vi "Close.vi"(6 "Priority (F)":bool, 8 "error in (no error)":errorcluster, 11 "Data":variant) -> (0 "error out":errorcluster)   [LabVIEW 2020, in "Controller.lvlib"]
uses:
  Private Controls/Element.ctl
  Private Controls/Module Action.ctl
  Controller.lvlib
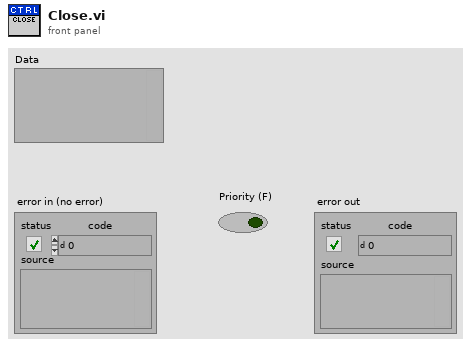
[diagram p1: front panel]
types:
  T1 = typedef "Controller.lvlib/Module Action.ctl" = enum16{"Initialise Module", "Connect", "Setup", "Pause", "Start", "Search Network", "Get Local", "Process Results", "Stop", "Show Match", "Show Full", "Get UI Refs", "Wait: Time Elapsed", "Error", "Exit"}
  T2 = typedef "Controller.lvlib/Element.ctl" = cluster{"Action":T1, "Data":variant}
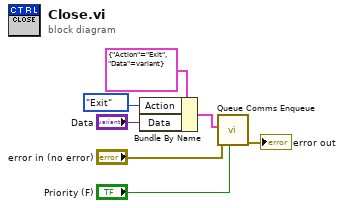
[diagram p0: block diagram]
diagram:
  n1 = Bundle By Name(cluster=T2 {"Action"=enum."Exit", "Data"=variant} ("Element"), "Action"=Module_Action."Exit", "Data"="Data") -> (w1:T2)
  n2 = call "Queue Comms Enqueue.vi"("Priority (F)"="Priority (F)", "error in (no error)"="error in (no error)", "Element"=w1) -> ("error out"=→"error out":errorcluster)  [unwired: 8 in]
